vi "Get Report Type.vi"(0 "report in":refnum<class "NI_HTML.lvclass">, 11 "error in (no error)":errorcluster) -> (4 "report out":refnum<class "NI_HTML.lvclass">, 8 "report type":T1(ring)=enum."HTML", 15 "error out":errorcluster)   [LabVIEW 2017, in "NI_HTML.lvclass"]
doc: "Returns the report type, such as standard, HTML, Word, or Excel, of a specified report."
uses:
  <vilib>/Utility/NIReport.llb/HTML/NI_HTML.lvclass
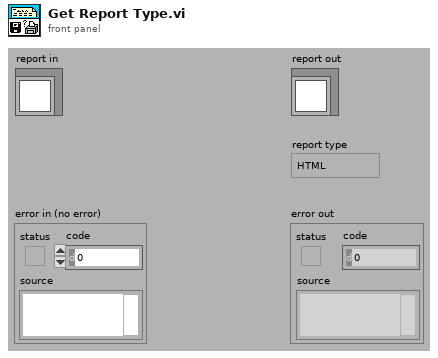
[diagram p1: front panel]
types:
  T1 = enum16{"Standard Report", "HTML", "Word", "Excel"}
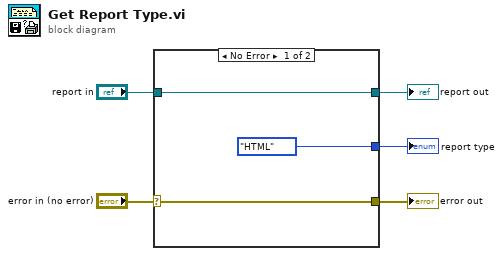
[diagram p0: block diagram]
diagram:
  n1 = case shown="No Error" "error in (no error)" {
    selector: "error in (no error)" -> [w8 w10]
    tunnel: [w8 w10] -> w4
    tunnel: [w7 w9] -> w2
    tunnel: "report in" -> [w7 w9]
    tunnel: [T1."HTML" ("output element") _] -> w1
    frame No Error {
    }
    frame Error {
    }
  }
  "error out" <- w4
  "report out" <- w2
  "report type" <- w1
